vi "WaitForAnyVI.vi"(8 "error in (no error)":errorcluster, 10 "Message_command In":T1={"No. of command"=14, "Parameters"=["BLM_ManualControl.vi", "BLM Position", "Within ", "10300", "10 min"], "Address"="", "Boolean"=TRUE, "No. of line"=159, "Initial Time"=timestamp(3580981392.875361 s since 1904-01-01), "Current Time"=timestamp(0 s since 1904-01-01), "Status"="Wait for VI value ", "Sequence Ref."=refnum, "Temp check"=0, "Sequence_History"="Set Parameter BLM_ManualControl.vi, New position, 10300, Number\rSet Parameter BLM_ManualControl.vi, Run, 1, Boolean\r", "Subsequence"=[]}, 11 "Command Queue In":T2) -> (0 "error out":errorcluster, 2 "Message_command Out":T1={"No. of command"=14, "Parameters"=["BLM_ManualControl.vi", "BLM Position", "Within ", "10300", "10 min"], "Address"="", "Boolean"=TRUE, "No. of line"=159, "Initial Time"=timestamp(3580981392.875361 s since 1904-01-01), "Current Time"=timestamp(0 s since 1904-01-01), "Status"="Wait for BLM_ManualControl.vi BLM Position value 0.0000  Within  10300 \nTime out: 10 min \nElapsed Time: 600.1013 sec", "Sequence Ref."=refnum, "Temp check"=0, "Sequence_History"="Set Parameter BLM_ManualControl.vi, New position, 10300, Number\rSet Parameter BLM_ManualControl.vi, Run, 1, Boolean\r", "Subsequence"=[]}, 3 "Command Queue out":T2)   [LabVIEW 2020]
uses:
  Command_Queue.ctl
  Command_Message.ctl
panel:
  out "resulting string":string
  out "x = y?":bool
  out "element":string
  in  "send timeout error?":bool=TRUE
  in  "in range window":dbl=0.01
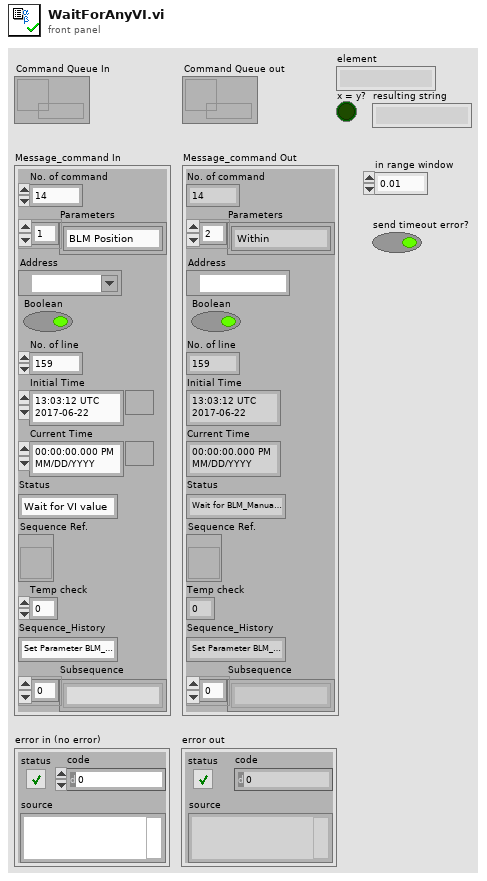
[diagram p1: front panel]
types:
  T1 = typedef "Command_Message.ctl" = cluster{"No. of command":i32, "Parameters":string[], "Address":refnum<visa-resource-name>, "Boolean":bool, "No. of line":i32, "Initial Time":timestamp, "Current Time":timestamp, "Status":string, "Sequence Ref.":refnum<vi>, "Temp check":i32, "Sequence_History":string, "Subsequence":string[]}
  T2 = typedef "Command_Queue.ctl" = refnum<queue>
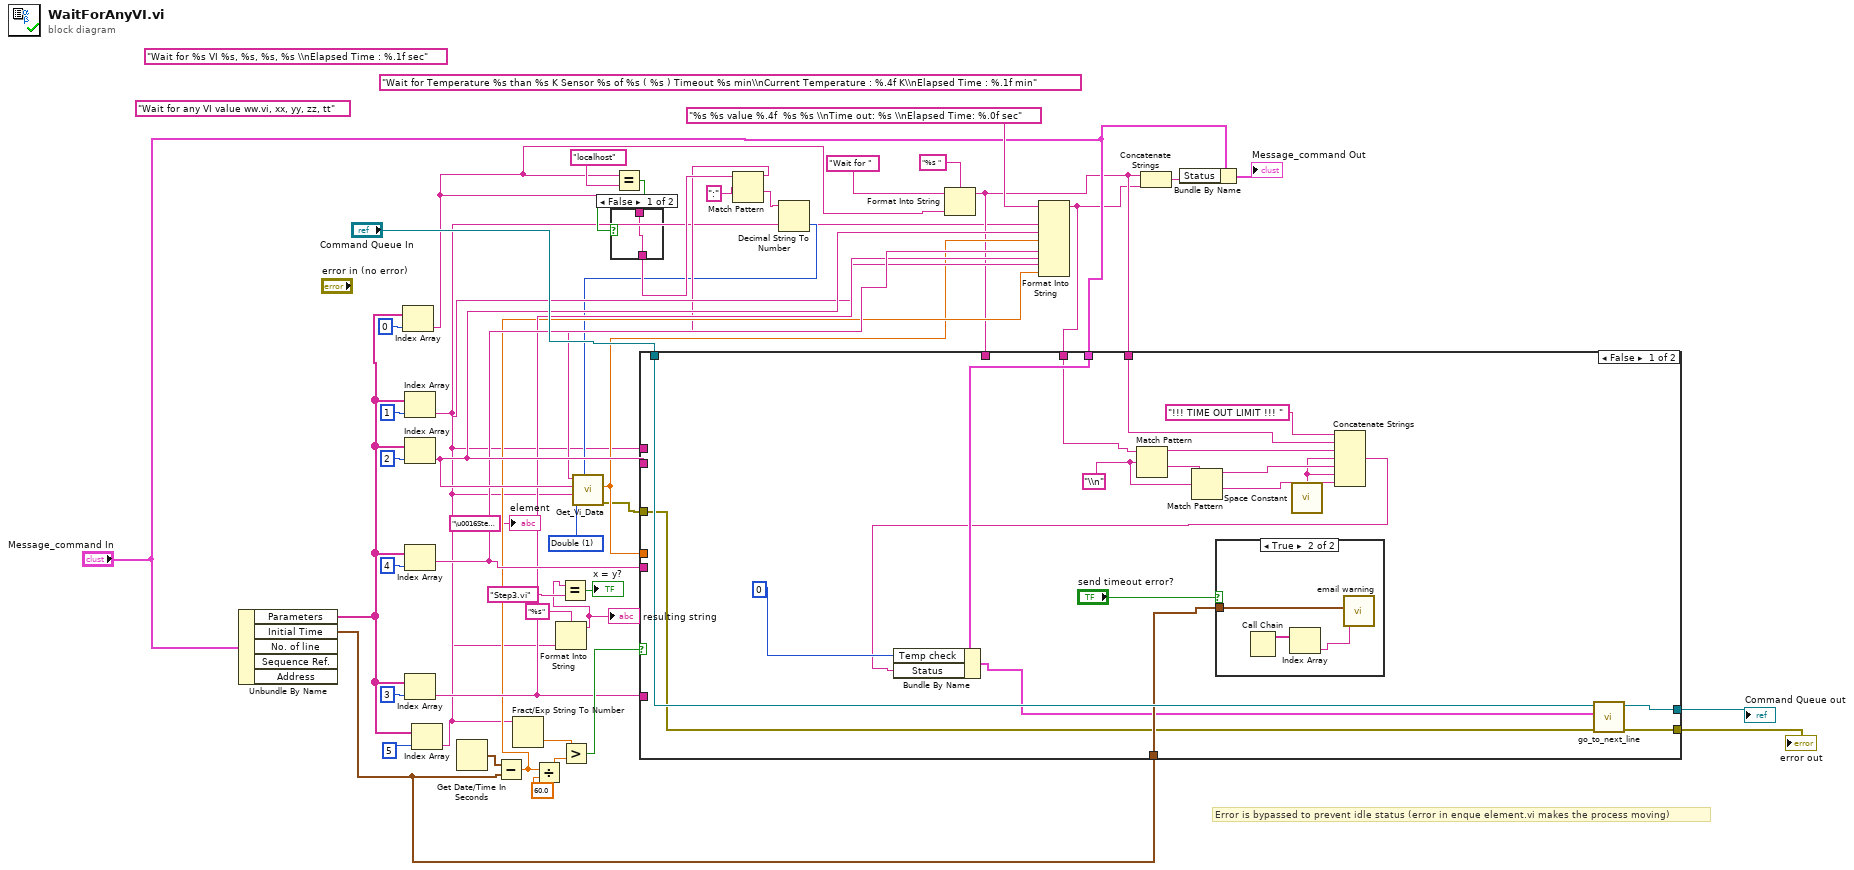
[diagram p0: block diagram]
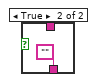
[diagram p2: hidden frame]
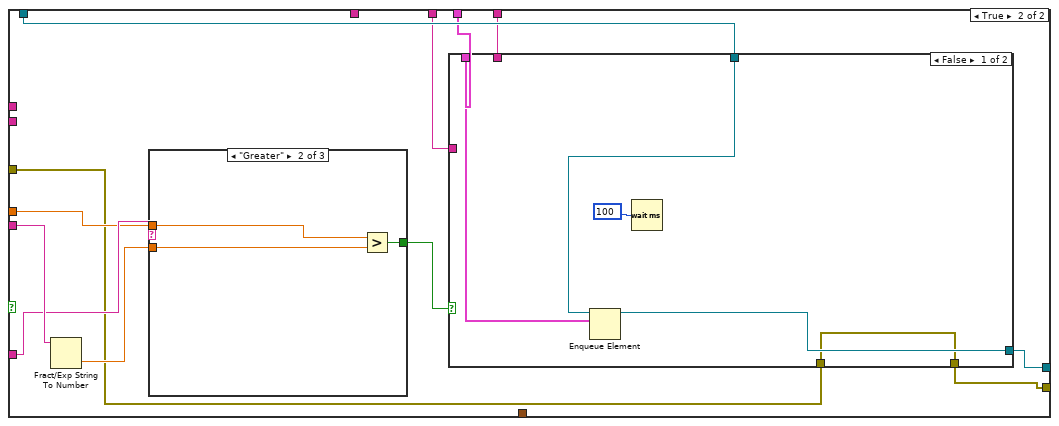
[diagram p4: hidden frame]
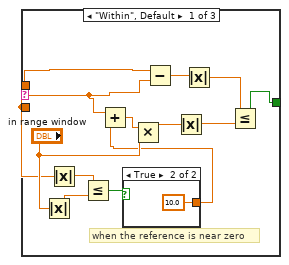
[diagram p5: hidden frame]
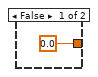
[diagram p6: hidden frame]
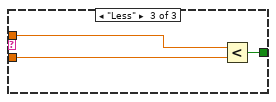
[diagram p7: hidden frame]
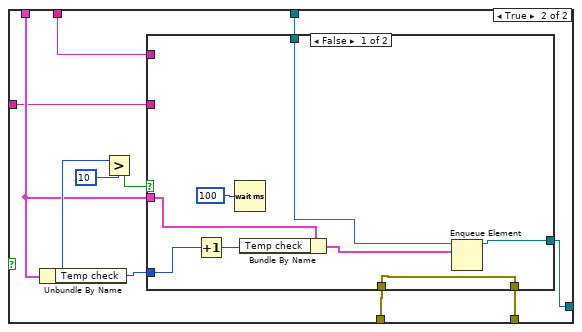
[diagram p8: hidden frame]
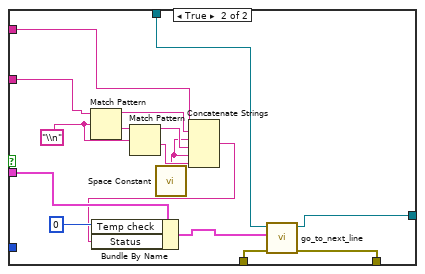
[diagram p9: hidden frame]
diagram:
  (unwired) "\u0016Step3.vi" ("element")
  w13 = u16 1 items=["String", "Double", "Boolean", "Variant"] ("Data Type")
  (unwired) "Wait for Temperature %s than %s K Sensor %s of %s ( %s ) Timeout %s min\\nCurrent Temperature : %.4f K\\nElapsed Time : %.1f min"
  (unwired) "Wait for any VI value ww.vi, xx, yy, zz, tt" ("format string")
  (unwired) "Wait for %s VI %s, %s, %s, %s \\nElapsed Time : %.1f sec" ("format string")
  # "Error is bypassed to prevent idle status (error in enque element.vi makes the process moving)"
  n1 = Unbundle By Name("Message_command In") -> ("Parameters"=w25:string[], "Initial Time"=w27:timestamp)  [unwired: 3 out]
  n2 = Index Array(array=w25, index=0) -> (element=w14:string)
  n3 = Index Array(array=w25, index=1) -> (element=w1:string)
  "element" <- w1
  n4 = Index Array(array=w25, index=2) -> (element=w32:string)
  n5 = Index Array(array=w25, index=4) -> (element=w31:string)
  n6 = Index Array(array=w25, index=3) -> (element=w30:string)
  n7 = Index Array(array=w25, index=5) -> (element=w28:string)
  n8 = Get Date/Time In Seconds() -> (seconds since 1Jan1904=w39:timestamp)
  n9 = Subtract(x=w39, y=w27) -> (x-y=w29:dbl)
  n10 = Fract/Exp String To Number(string=w28) -> (number=w38:dbl)  [unwired: 3 in, 1 out]
  n11 = Divide(x=w29, y=60.0) -> (x/y=w37:dbl)
  n12 = Format Into String(format string="%s", w1) -> (resulting string=w2:string)  [unwired: 2 in, 1 out]
  "resulting string" <- w2
  n13 = Equal?(x=w2, y="Step3.vi") -> (x = y?=→"x = y?":bool)
  n14 = Greater?(x=w38, y=w37) -> (0:w36:bool)
  n15 = Equal?(x=w14, y="localhost") -> (x = y?=w18:bool)
  n16 = case shown="False" w18 {
    tunnel: [w46 ""] -> w17
    tunnel: w14 -> [w46 _]
    frame False {
    }
    frame True {
    }
  }
  n17 = Match Pattern(string=w17, regular expression=":") -> (before substring=w16:string, after substring=w20:string)  [unwired: 1 in, 2 out]
  n18 = Decimal String To Number(string=w20) -> (number=w15:i32)  [unwired: 2 in, 1 out]
  n19 = call "Get_Vi_Data.vi"("port number"=w15, "Data Type"=w13, "VI name"=w1, "Control Name"=w32, "Data mac ip address"=w16) -> ("error out"=w7:errorcluster, "Data (Double)"=w12:dbl)  [unwired: 2 in, 3 out]
  n20 = Format Into String(format string="%s ", initial string="Wait for " ("format string"), w14) -> (resulting string=w9:string)  [unwired: 1 in, 1 out]
  n21 = Format Into String(format string="%s %s value %.4f  %s %s \\nTime out: %s \\nElapsed Time: %.0f sec", w1, w32, w12, w30, w31, w28, w29) -> (resulting string=w8:string)  [unwired: 2 in, 1 out]
  n22 = case shown="False" w36 {
    tunnel: w1 -> [_ _]
    tunnel: w32 -> [_ _]
    tunnel: w31 -> [_ w81]
    tunnel: w30 -> [_ w76]
    tunnel: "Message_command In" -> [w63 w74]
    tunnel: "Command Queue In" -> [w65 w80]
    tunnel: [w64 w79] -> w34
    tunnel: w27 -> [w62 _]
    tunnel: w12 -> [_ w75]
    tunnel: w9 -> [_ _]
    tunnel: w9 -> [w57 w73]
    tunnel: w8 -> [w56 w72]
    tunnel: w7 -> [w49 w71]
    tunnel: [w48 w70] -> w6
    frame False {
      w60 = "\\n"
      n23 = Match Pattern(string=w56, regular expression=w60) -> (before substring=w59:string, after substring=w58:string)  [unwired: 1 in, 2 out]
      n24 = Match Pattern(string=w58, regular expression=w60) -> (before substring=w51:string, after substring=w52:string)  [unwired: 1 in, 2 out]
      n25 = case shown="True" "send timeout error?" {
        tunnel: w62 -> [_ w69]
        frame False {
        }
        frame True {
          n26 = Call Chain() -> (call chain=w68:string[])
          n27 = Index Array(array=w68) -> (element=w67:string)  [unwired: 1 in]
          n28 = call "email warning.vi"("running VI"=w67, "Initial"=w69) -> ()  [unwired: 9 in, 1 out]
        }
      }
      n29 = call <vilib>:"Space Constant.vi"() -> ("String"=w50:string)
      n30 = Concatenate Strings("!!! TIME OUT LIMIT !!! " ("string"), w57, w59, w50, w51, w50, w52) -> (w54:string)
      n31 = Bundle By Name(cluster=w63, "Temp check"=0, "Status"=w54) -> (w53:T1)
      n32 = call "go_to_next_line.vi"("error in (no error)"=w49, "Message_command in"=w53, "Command Queue in"=w65) -> ("error out"=w48:errorcluster, "Command Queue out"=w64:T2)  [unwired: 7 in]
    }
    frame True {
      n33 = Fract/Exp String To Number(string=w81) -> (number=w78:dbl)  [unwired: 3 in, 1 out]
      n34 = case shown="\"Greater\"" w76 {
        tunnel: w75 -> [w86 w99 w102]
        tunnel: w78 -> [w84 w98 w101]
        tunnel: [w91 w97 w100] -> w77
        frame "Within", Default {
          # "when the reference is near zero"
          n35 = Absolute Value(x="in range window") -> (abs(x)=w87:dbl)
          n36 = Absolute Value(x=w84) -> (abs(x)=w88:dbl)
          n37 = Less Or Equal?(x=w88, y=w87) -> (x <= y?=w89:bool)
          n38 = case shown="True" w89 {
            tunnel: [0.0 ("in range window") 10.0 ("in range window")] -> w83
            frame False {
            }
            frame True {
            }
          }
          n39 = Add(x=w84, y=w83) -> (x+y=w85:dbl)
          n40 = Multiply(x=w85, y="in range window") -> (x*y=w93:dbl)
          n41 = Subtract(x=w86, y=w84) -> (x-y=w94:dbl)
          n42 = Absolute Value(x=w93) -> (abs(x)=w92:dbl)
          n43 = Absolute Value(x=w94) -> (abs(x)=w82:dbl)
          n44 = Less Or Equal?(x=w82, y=w92) -> (x <= y?=w91:bool)
        }
        frame "Greater" {
          n45 = Greater?(x=w99, y=w98) -> (0:w97:bool)
        }
        frame "Less" {
          n46 = Less?(x=w102, y=w101) -> (x < y?=w100:bool)
        }
      }
      n47 = case shown="False" w77 {
        tunnel: w74 -> [w105 w114]
        tunnel: w80 -> [w106 w113]
        tunnel: [w104 w112] -> w79
        tunnel: w73 -> [_ w111]
        tunnel: w72 -> [_ w110]
        tunnel: w71 -> [w103 w109]
        tunnel: [w103 w108] -> w70
        frame False {
          n48 = Enqueue Element(queue=w106, element=w105) -> (queue out=w104:T2)  [unwired: 2 in, 2 out]
          n49 = Wait (ms)(milliseconds to wait=u32 100) -> ()  [unwired: 1 out]
        }
        frame True {
          n50 = Unbundle By Name(w114) -> ("Temp check"=w115:i32)
          n51 = Greater?(x=w115, y=10) -> (0:w116:bool)
          n52 = case shown="False" w116 {
            tunnel: [w124 w141] -> w112
            tunnel: w115 -> [w122 _]
            tunnel: w114 -> [w120 w139]
            tunnel: w113 -> [w119 w138]
            tunnel: w111 -> [_ w133]
            tunnel: w110 -> [_ w134]
            tunnel: w109 -> [w118 w127]
            tunnel: [w118 w126] -> w108
            frame False {
              n53 = Increment(x=w122) -> (x+1=w125:i32)
              n54 = Wait (ms)(milliseconds to wait=u32 100) -> ()  [unwired: 1 out]
              n55 = Bundle By Name(cluster=w120, "Temp check"=w125) -> (w121:T1)
              n56 = Enqueue Element(queue=w119, element=w121) -> (queue out=w124:T2)  [unwired: 2 in, 2 out]
            }
            frame True {
              w137 = "\\n"
              n57 = Match Pattern(string=w134, regular expression=w137) -> (before substring=w136:string, after substring=w135:string)  [unwired: 1 in, 2 out]
              n58 = Match Pattern(string=w135, regular expression=w137) -> (before substring=w129:string, after substring=w130:string)  [unwired: 1 in, 2 out]
              n59 = call <vilib>:"Space Constant.vi"() -> ("String"=w128:string)
              n60 = Concatenate Strings(w133, w136, w128, w129, w128, w130) -> (w132:string)
              n61 = Bundle By Name(cluster=w139, "Temp check"=0, "Status"=w132) -> (w131:T1)
              n62 = call "go_to_next_line.vi"("error in (no error)"=w127, "Message_command in"=w131, "Command Queue in"=w138) -> ("error out"=w126:errorcluster, "Command Queue out"=w141:T2)  [unwired: 7 in]
            }
          }
        }
      }
    }
  }
  "Command Queue out" <- w34
  "error out" <- w6
  n63 = Concatenate Strings(w9, w8) -> (w22:string)
  n64 = Bundle By Name(cluster="Message_command In", "Status"=w22) -> (→"Message_command Out":T1)
